vi "Vision Processing.vi"() -> ()   [LabVIEW 2011]
doc: "This VI runs in parallel to other tasks. It gets images from the camera, processes them for color or shape and use that information to affect robot behavior."
uses:
  <vilib>/Rock Robotics/WPI/Camera/WPI_CameraWhite Balance Values.ctl
  Robot Global Data.vi
  <vilib>/vision/NI_Vision_Development_Module.lvlib
panel:
  out "Y Position Array":dbl[][](array[numeric])
  out "X Position Array":dbl[][](array[numeric])
  out "Processed Image":T1(plugin-control)
  out "Original Image":T1(plugin-control)
  in  "Annotate":bool=TRUE
  in  "Particle Count Limit":i32=10
  in  "Area Size Limit":i32=444
  in  "Range":cluster{"Lower value":sgl, "Upper value":sgl}={"Lower value"=120.0, "Upper value"=255.0}
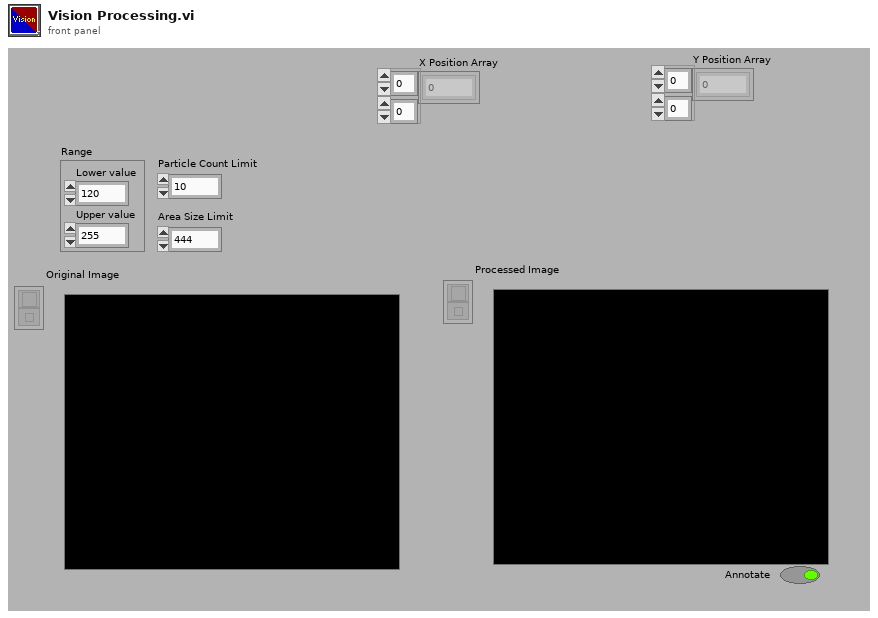
[diagram p1: front panel]
types:
  T1 = typedef "IMAQ Image.ctl" = refnum<image>
  T2 = typedef "WPI_CameraWhite Balance Values.ctl" = enum16{"Auto", "Fixed indoor", "Fixed outdoor 1", "Fixed outdoor 2", "Fixed fluorescent 1", "Fixed fluorescent 2", "Hold current"}
  T3 = typedef "Image Type" = u32
  T4 = typedef "WPI_CameraImageSize.ctl" = enum16{"640x480", "320x240", "160x120"}
  T5 = cluster{"fps":i32, "compression":i32, "Image Size":T4}
  T6 = typedef "WPI_CameraDevRef.ctl" = cluster{"Camera Address":string, "CameraStatus":errorcluster, "Acquire Image Notifier":refnum<notifier>}
  T7 = cluster{"Rect Coverage":dbl, "Aspect Ratio":dbl, "X Edge Strength":dbl, "Y Edge Strength":dbl}
  T8 = cluster{"Position":cluster{"X":dbl, "Y":dbl}, "Distance (ft)":dbl}[]
  T9 = cluster{cluster{"Left":dbl, "Top":dbl, "Right":dbl, "Bottom":dbl}, dbl[]}[]
  T10 = cluster{"Left":dbl, "Top":dbl, "Right":dbl, "Bottom":dbl}
  T11 = cluster{"Target Center (-1 to 1)":cluster{"X":dbl, "Y":dbl}, "Distance (ft)":dbl}
  T12 = cluster{"Target Center (-1 to 1)":cluster{"X":dbl, "Y":dbl}, "Distance (ft)":dbl}[]
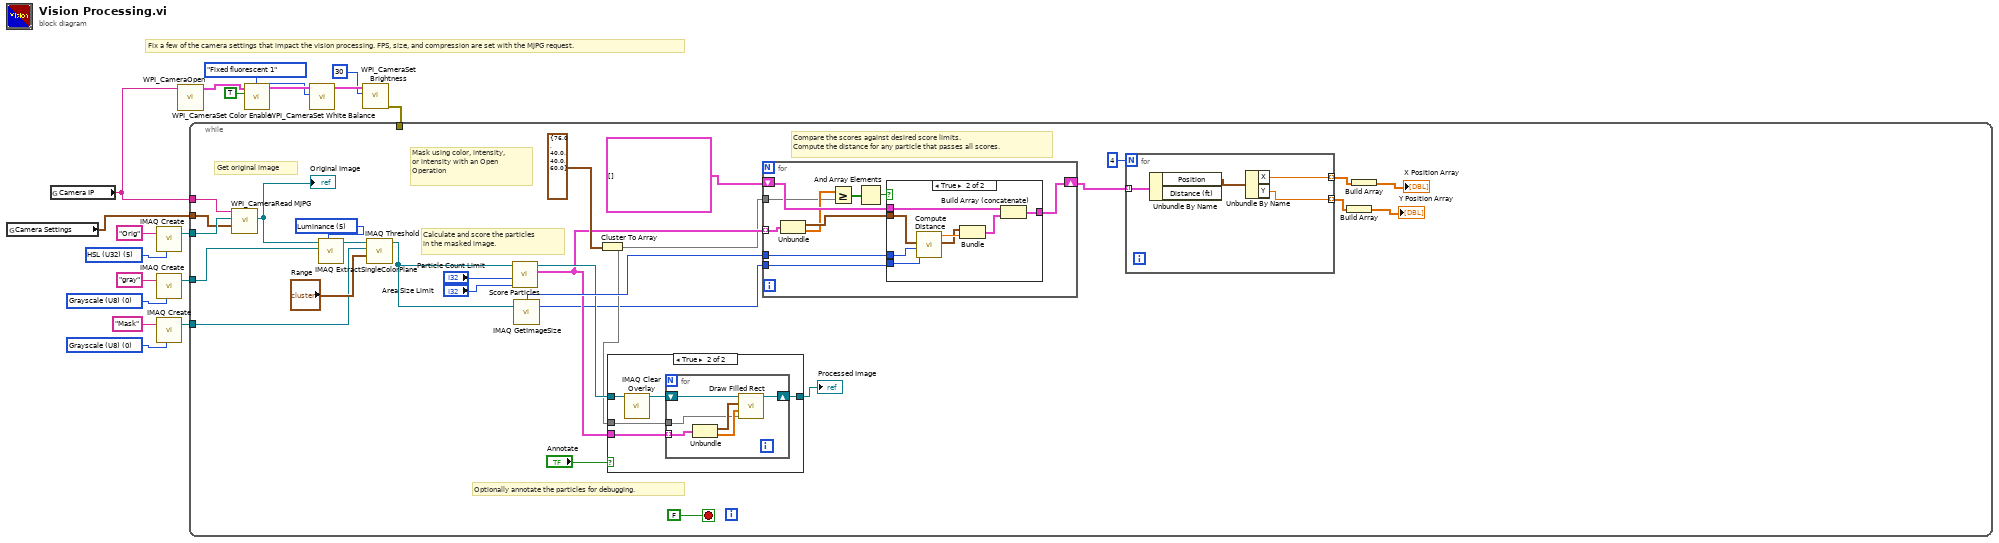
[diagram p0: block diagram]
diagram:
  w11 = T3 0 items=["Grayscale (U8)", "Grayscale (I16)", "Grayscale (SGL)", "Complex (CSG)", "RGB (U32)", "HSL (U32)", "RGB (U64)", "Grayscale (U16)"] ("Image Type")
  w15 = T3 5 items=["Grayscale (U8)", "Grayscale (I16)", "Grayscale (SGL)", "Complex (CSG)", "RGB (U32)", "HSL (U32)", "RGB (U64)", "Grayscale (U16)"] ("Image Type")
  w18 = T3 0 items=["Grayscale (U8)", "Grayscale (I16)", "Grayscale (SGL)", "Complex (CSG)", "RGB (U32)", "HSL (U32)", "RGB (U64)", "Grayscale (U16)"] ("Image Type")
  # "Fix a few of the camera settings that impact the vision processing. FPS, size, and compression are set with the MJPG request."
  n1 = global read "Robot Global Data.vi" "Camera Settings"() -> (w1:T5)
  n2 = global read "Robot Global Data.vi" "Camera IP"() -> (w2:string)
  n3 = call "IMAQ Create"("Image Name"="Orig", "Image Type"=w15) -> ("New Image"=w14:T1)  [unwired: 2 in, 2 out]
  n4 = call "IMAQ Create"("Image Name"="gray", "Image Type"=w18) -> ("New Image"=w13:T1)  [unwired: 2 in, 2 out]
  n5 = call "IMAQ Create"("Image Name"="Mask", "Image Type"=w11) -> ("New Image"=w10:T1)  [unwired: 2 in, 2 out]
  n6 = call <vilib>:"WPI_CameraOpen.vi"("Camera Address"=w2) -> ("CameraDevRef"=w9:T6)  [unwired: 9 in, 1 out]
  n7 = call <vilib>:"WPI_CameraSet Color Enable.vi"("Color Enabled"=TRUE, "CameraDevRef"=w9) -> ("CameraDevRef Out"=w7:T6)  [unwired: 8 in, 1 out]
  n8 = call <vilib>:"WPI_CameraSet White Balance.vi"("White Balance"=WPI_CameraWhite_Balance_Values."Fixed fluorescent 1", "CameraDevRef"=w7) -> ("CameraDevRef Out"=w5:T6)  [unwired: 8 in, 1 out]
  n9 = call <vilib>:"WPI_CameraSet Brightness.vi"("Brightness"=30, "CameraDevRef"=w5) -> ("error out"=w3:errorcluster)  [unwired: 8 in, 1 out]
  n10 = while {
    tunnel: w14 -> [w44]
    tunnel: w13 -> [w26]
    tunnel: w10 -> [w28]
    tunnel: w2 -> [w43]
    tunnel: w3 -> [_]
    tunnel: w1 -> [w32]
    stop <- FALSE stop-if-true
    w31 = 5 items=["Red", "Green", "Blue", "Hue", "Saturation", "Luminance", "Value", "Intensity"] ("Color Plane")
    # "Optionally annotate the particles for debugging."
    # "Compare the scores against desired score limits.\nCompute the distance for any particle that passes all scores."
    # "Calculate and score the particles\nin the masked image."
    # "Mask using color, intensity,\nor intensity with an Open\nOperation"
    # "Get original image"
    n11 = call <vilib>:"WPI_CameraRead MJPG.vi"("Camera Settings"=w32, "Image"=w44, "address"=w43) -> ("Image Out"=w27:T1)  [unwired: 7 in, 1 out]
    "Original Image" <- w27
    n12 = call "IMAQ ExtractSingleColorPlane"("Color Plane"=w31, "Image Dst"=w26, "Image Src"=w27) -> ("Image Dst Out"=w29:T1)  [unwired: 1 in, 7 out]
    n13 = call "IMAQ Threshold"("Range"="Range", "Image Dst"=w28, "Image Src"=w29) -> ("Image Dst Out"=w25:T1)  [unwired: 3 in, 5 out]
    n14 = call "Score Particles.vi"("Area Size Limit"="Area Size Limit", "Particle Count Limit"="Particle Count Limit", "Image Refnum in"=w25) -> ("Scored Particle Info"=w39:T9, "Image Refnum out"=w42:T1)  [unwired: 7 in]
    n15 = call "IMAQ GetImageSize"("Image"=w25) -> ("Y Resolution"=w33:i32, "X Resolution"=w45:i32)  [unwired: 3 in, 1 out]
    n16 = Cluster To Array(cluster=T7 {"Rect Coverage"=76.0, "Aspect Ratio"=40.0, "X Edge Strength"=40.0, "Y Edge Strength"=60.0} ("Score Limits")) -> (array=w37:dbl[])
    n17 = case shown="True" "Annotate" {
      tunnel: w42 -> [w51 w56]
      tunnel: [w51 w55] -> w40
      tunnel: w39 -> [_ w53]
      tunnel: w37 -> [_ w52]
      frame False {
      }
      frame True {
        n18 = call "IMAQ Clear Overlay"("Image"=w56) -> ("Image Out"=w54:T1)  [unwired: 2 in, 8 out]
        n19 = for {
          shift-right: [w61] -> w55
          shift-left: w54 -> [w62]
          tunnel: w53 -> [w58] mode=indexing
          tunnel: w52 -> [w57]
          n20 = Unbundle(w58) -> (w59:T10, w60:dbl[])
          n21 = call "Draw Filled Rect.vi"("Limits"=w57, "Scores"=w60, "Bounding Box"=w59, "image in"=w62) -> ("image out"=w61:T1)  [unwired: 7 in]
        }
      }
    }
    "Processed Image" <- w40
    n22 = for {
      shift-right: [w71] -> w23
      shift-left: T8 [] -> [w72]
      tunnel: w45 -> [w70]
      tunnel: w39 -> [w68] mode=indexing
      tunnel: w37 -> [w64]
      tunnel: w33 -> [w63]
      n23 = Unbundle(w68) -> (w69:T10, w65:dbl[])
      n24 = Greater Or Equal?(x=w65, y=w64) -> (x >= y?=w67:bool[])
      n25 = And Array Elements(Boolean array=w67) -> (logical AND=w66:bool)
      n26 = case shown="True" w66 {
        tunnel: w72 -> [w73 w81]
        tunnel: [w73 w80] -> w71
        tunnel: w69 -> [_ w76]
        tunnel: w70 -> [_ w78]
        tunnel: w63 -> [_ w74]
        frame False {
        }
        frame True {
          n27 = call "Compute Distance.vi"("Y Image Resolution"=w74, "X Image Resolution"=w78, "Bounding Box"=w76) -> ("Target Center (-1 to 1)"=w75:cluster{"X":dbl, "Y":dbl}, "Distance (ft)"=w77:dbl)  [unwired: 7 in]
          n28 = Bundle("Target Center (-1 to 1)"=w75, "Distance (ft)"=w77) -> (w79:T11)  [unwired: 1 in]
          n29 = Build Array (concatenate)(w81, w79) -> (w80:T12)
        }
      }
    }
    n30 = for {
      N: 4 -> [_]
      tunnel: w23 -> [w50] mode=indexing
      tunnel: [w48] -> w22 mode=indexing
      tunnel: [w47] -> w19 mode=indexing
      n31 = Unbundle By Name(w50) -> ("Position"=w49:cluster{"X":dbl, "Y":dbl})  [unwired: 1 out]
      n32 = Unbundle By Name(w49) -> ("X"=w48:dbl, "Y"=w47:dbl)
    }
    n33 = Build Array(w19) -> (→"Y Position Array":dbl[][])
    n34 = Build Array(w22) -> (→"X Position Array":dbl[][])
  }
